vi "set control parameters.vi"(6 "Control slope limit (10 V/min)":dbl[unit]=0.16666666666666666, 7 "Proportional (10)":dbl=10.0, 8 "error in (no error)":errorcluster, 9 "Ramp rate (3500 Gs/min)":dbl[unit]=0.005833333333333334, 10 "Integral (1 s)":dbl[unit]=1.0, 11 "VISA session":refnum<visa-resource-name>) -> (0 "error out":errorcluster, 3 "dup VISA session":refnum<visa-resource-name>)   [LabVIEW 2017]
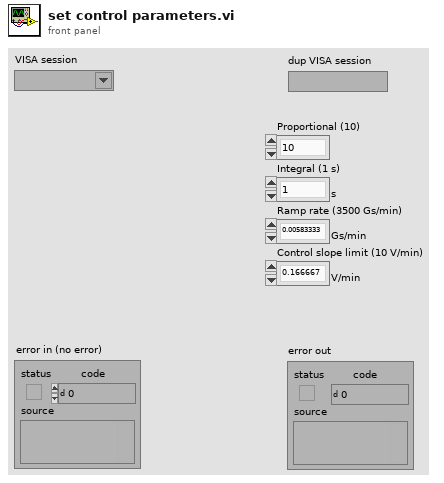
[diagram p1: front panel]
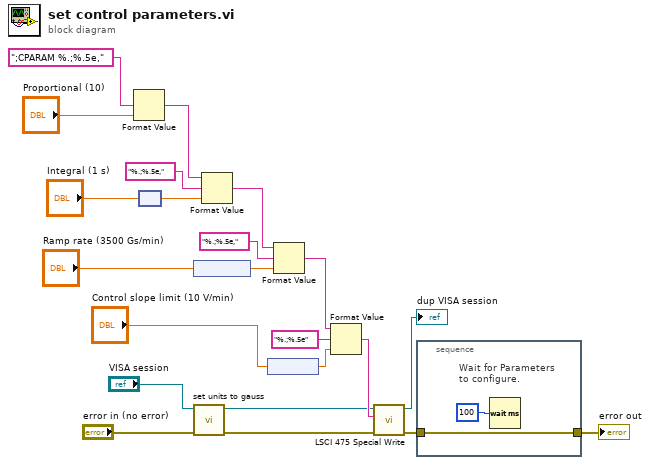
[diagram p0: block diagram]
diagram:
  n1 = Format Value(format string=";CPARAM %.;%.5e,", value (0)="Proportional (10)") -> (output string=w17:string)  [unwired: 1 in]
  n2 = node("Integral (1 s)") -> (w5:dbl)
  n3 = node("Ramp rate (3500 Gs/min)") -> (w3:dbl)
  n4 = call "set units to gauss.vi"("VISA session"="VISA session", "error in (no error)"="error in (no error)") -> ("dup VISA session"=w10:refnum<visa-resource-name>, "error out"=w8:errorcluster)  [unwired: 7 in]
  n5 = Format Value(string ("")=w17, format string="%.;%.5e,", value (0)=w5) -> (output string=w16:string)
  n6 = node("Control slope limit (10 V/min)") -> (w2:dbl)
  n7 = Format Value(string ("")=w16, format string="%.;%.5e,", value (0)=w3) -> (output string=w15:string)
  n8 = Format Value(string ("")=w15, format string="%.;%.5e", value (0)=w2) -> (output string=w12:string)
  n9 = call "LSCI 475 Special Write.vi"("error in (no error)"=w8, "Write Buffer (\"\")"=w12, "VISA session"=w10) -> ("error out"=w14:errorcluster, "dup VISA session"=→"dup VISA session":refnum<visa-resource-name>)  [unwired: 6 in, 1 out]
  n10 = stacked-sequence {
    tunnel: w14 -> [w23]
    tunnel: [w23] -> w13
    frame #0 {
      # "Wait for Parameters\nto configure."
      n11 = Wait (ms)(milliseconds to wait=u32 100) -> ()  [unwired: 1 out]
    }
  }
  "error out" <- w13
